vi "Item Modify.vi"(0 "Tree Reference In":refnum<vi>, 1 "Tag to Modify (Current)":string, 2 "New Tag Value (No Change)":string, 3 "New Text Value (No Change)":string, 4 "Element Data":variant, 5 "error in (no error)":errorcluster, 7 "Symbol(-1:No Change)":i32=-1, 9 "Column # (0)":i32) -> (14 "Tree Reference Out":refnum<vi>, 16 "Tag Value out":string, 19 "error out":errorcluster)   [LabVIEW 2013, in "QuickVIew.lvlib"]
doc: "Modifies an item in the tree. Uses the current item if input is blank. Allows to modify both the tag and text"
uses:
  QuickVIew.lvlib
  Typedef/TYPEDEF - DataStore Command.ctl
panel:
  # "VI INPUTS"
  # "VI OUTPUTS"
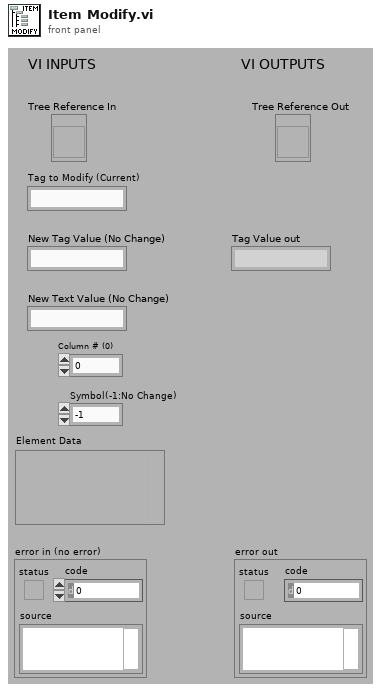
[diagram p1: front panel]
types:
  T1 = typedef "QuickVIew.lvlib/TYPEDEF - DataStore Command.ctl" = enum16{"Init", "Add", "Get", "Clear Tree", "Clear All", "Modify"}
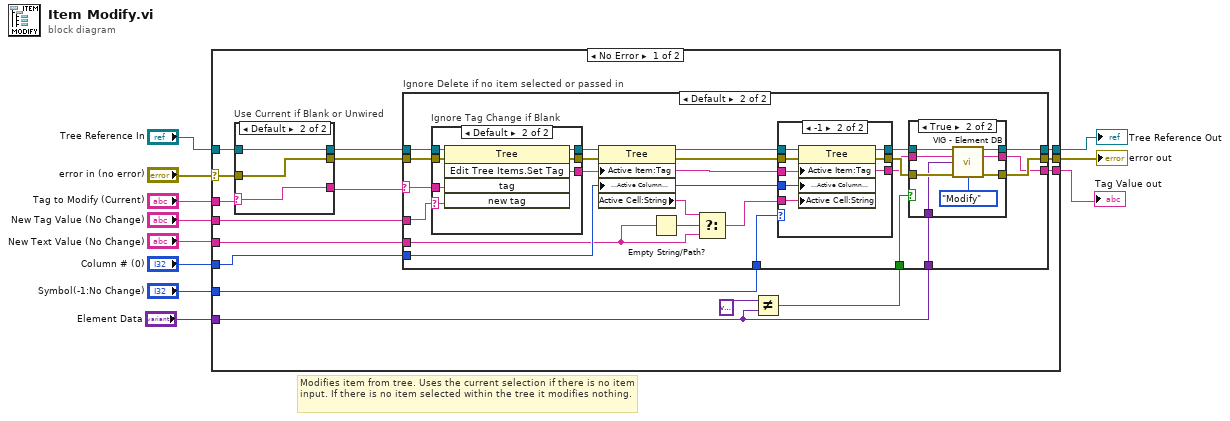
[diagram p0: block diagram]
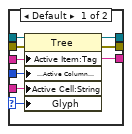
[diagram p4: hidden frame]
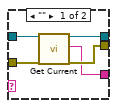
[diagram p6: hidden frame]
diagram:
  # "Modifies item from tree. Uses the current selection if there is no item input. If there is no item selected within the tree it modifies nothing."
  n1 = case shown="No Error" "error in (no error)" {
    selector: "error in (no error)" -> [w25 w99]
    tunnel: "Tree Reference In" -> [w27 w100]
    tunnel: [w24 w100] -> w10
    tunnel: [w23 w99] -> w9
    tunnel: "Tag to Modify (Current)" -> [w26 w98]
    tunnel: "New Text Value (No Change)" -> [w19 _]
    tunnel: "New Tag Value (No Change)" -> [w18 _]
    tunnel: "Column # (0)" -> [w17 _]
    tunnel: "Symbol(-1:No Change)" -> [w16 _]
    tunnel: [w15 w98] -> w2
    tunnel: "Element Data" -> [w13 _]
    frame No Error {
      n2 = case "Use Current if Blank or Unwired" shown="Default" w26 {
        selector: w26 -> [_ w95]
        tunnel: [w93 w97] -> w22
        tunnel: w27 -> [w94 w97]
        tunnel: [w92 w96] -> w21
        tunnel: w25 -> [w91 w96]
        tunnel: [w90 w95] -> w20
        frame "" {
          n3 = call "Get Current.vi"("Tree Reference In"=w94, "error in (no error)"=w91) -> ("Tree Reference Out"=w93:refnum<vi>, "Current Tag"=w90:string, "error out"=w92:errorcluster)  [unwired: 15 out]
        }
        frame Default {
        }
      }
      n4 = Not Equal?(x=variant ("Element Data"), y=w13) -> (x != y?=w12:bool)
      n5 = case "Ignore Delete if no item selected or passed in" shown="Default" w20 {
        selector: w20 -> [w28 w51]
        tunnel: [w30 w37] -> w24
        tunnel: [w29 w33] -> w23
        tunnel: w22 -> [w30 w52]
        tunnel: w21 -> [w29 w53]
        tunnel: w19 -> [_ w41]
        tunnel: w18 -> [_ w50]
        tunnel: w17 -> [_ w46]
        tunnel: w16 -> [_ w49]
        tunnel: [w28 w32] -> w15
        tunnel: w13 -> [_ w34]
        tunnel: w12 -> [_ w31]
        frame "" {
        }
        frame Default {
          n6 = case "Ignore Tag Change if Blank" shown="Default" w50 {
            selector: w50 -> [_ w83]
            tunnel: w53 -> [w81 w89]
            tunnel: [w81 w88] -> w43
            tunnel: w52 -> [w82 w87]
            tunnel: w51 -> [w80 w86]
            tunnel: [w80 w85] -> w45
            tunnel: [w82 w84] -> w44
            frame "" {
            }
            frame Default {
              n7 = invoke class="Tree" method="Edit Tree Items.Set Tag"(reference=w87, error in=w89, "tag"=w86, "new tag"=w83) -> (reference out=w84:refnum<vi>, error out=w88:errorcluster, "Edit Tree Items:Set Tag"=w85:string)  [unwired: 1 in, 2 out]
            }
          }
          n8 = property class="Tree"(reference=w44, error in=w43, "Active Item:Tag"=w45, "Active Cell:Active Column Number"=w46) -> (reference out=w40:refnum<vi>, error out=w39:errorcluster, "Active Cell:String"=w42:string)
          n9 = Empty String/Path?(string/path=w41) -> (empty?=w48:bool)
          n10 = Select(t=w42, s=w48, f=w41) -> (s? t:f=w47:string)
          n11 = case shown="-1" w49 {
            selector: w49 -> [w66 _]
            tunnel: w39 -> [w72 w79]
            tunnel: [w71 w78] -> w38
            tunnel: [w70 w77] -> w36
            tunnel: w45 -> [w65 w73]
            tunnel: w47 -> [w69 w76]
            tunnel: w40 -> [w68 w75]
            tunnel: w46 -> [w67 w74]
            tunnel: [w65 w73] -> w35
            frame Default {
              n12 = property class="Tree"(reference=w68, error in=w72, "Active Item:Tag"=w65, "Active Cell:Active Column Number"=w67, "Active Cell:String"=w69, "Glyph"=w66) -> (reference out=w71:refnum<vi>, error out=w70:errorcluster)
            }
            frame -1 {
              n13 = property class="Tree"(reference=w75, error in=w79, "Active Item:Tag"=w73, "Active Cell:Active Column Number"=w74, "Active Cell:String"=w76) -> (reference out=w78:refnum<vi>, error out=w77:errorcluster)
            }
          }
          n14 = case shown="True" w31 {
            tunnel: w38 -> [w54 w64]
            tunnel: [w54 w63] -> w37
            tunnel: w36 -> [w56 w62]
            tunnel: w35 -> [w55 w61]
            tunnel: w34 -> [_ w60]
            tunnel: [w56 w59] -> w33
            tunnel: [w55 w58] -> w32
            frame False {
            }
            frame True {
              n15 = call "VIG - Element DB.vi"("Tree Ref In"=w64, "Element Tag"=w61, "Tree Element Data In"=w60, "error in (no error)"=w62, "Command"=TYPEDEF_-_DataStore_Command."Modify") -> ("Tree Ref Out"=w63:refnum<vi>, "Element Tag Out"=w58:string, "error out"=w59:errorcluster)  [unwired: 8 out]
            }
          }
        }
      }
    }
    frame Error {
    }
  }
  "Tree Reference Out" <- w10
  "error out" <- w9
  "Tag Value out" <- w2
